vi "GetMicronArgs.vi"(8 "error in (no error)":errorcluster) -> (0 "error out":errorcluster, 3 "Micron Args":T1)   [LabVIEW 2019, in "MicronServer.lvlib" / "ServiceBase.lvclass"]
uses:
  ServiceBase.lvclass
  Typedefs/Micron Args.ctl
  <vilib>/SLL Toolkit/SLL String/_SubVIs/1D String Array to String.vi
  <vilib>/SLL Toolkit/SLL String/SLL String.lvlib
  <vilib>/regexp/Match Regular Expression.xnode
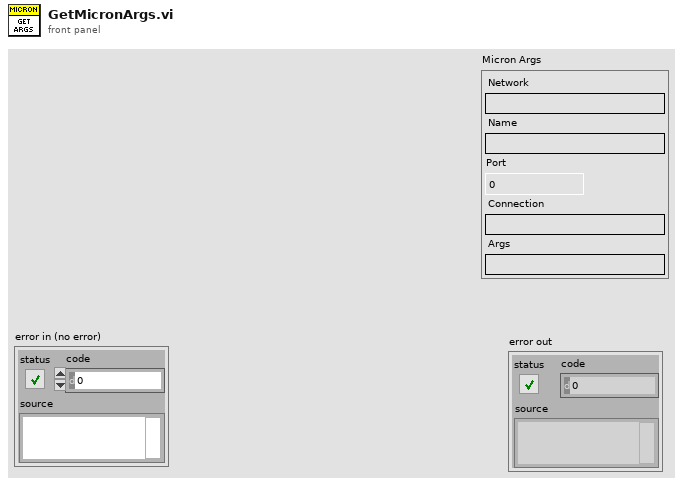
[diagram p1: front panel]
types:
  T1 = typedef "MicronServer.lvlib/ServiceBase.lvclass/Micron Args.ctl" = cluster{"Network":string, "Name":string, "Port":i32, "Connection":string, "Args":string}
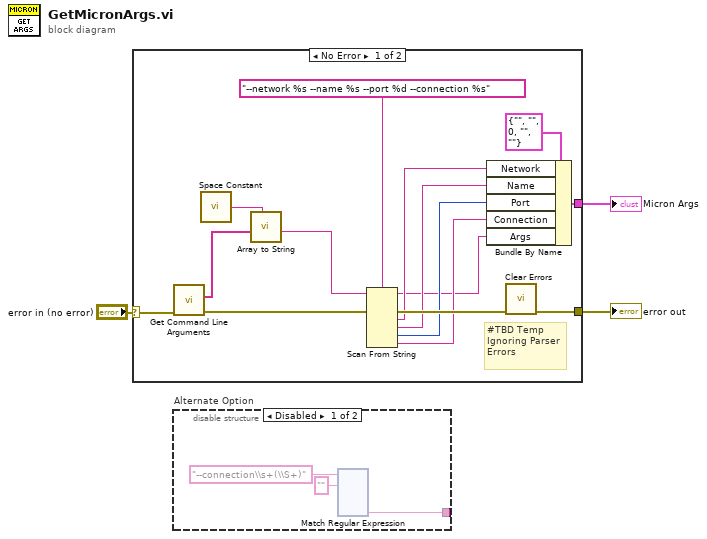
[diagram p0: block diagram]
diagram:
  n1 = case shown="No Error" "error in (no error)" {
    selector: "error in (no error)" -> [w18 w19]
    tunnel: [w4 w19] -> w2
    tunnel: [w5 _] -> w1
    frame No Error {
      # "#TBD Temp \nIgnoring Parser Errors"
      n2 = call <vilib>:"Get Command Line Arguments.vi"("error in (no error)"=w18) -> ("error out"=w15:errorcluster, "arguments"=w17:string[])  [unwired: 8 in, 1 out]
      n3 = call <vilib>:"Space Constant.vi"() -> ("String"=w16:string)
      n4 = call-poly <vilib>:"Array to String.vi"("Delimiter (,)"=w16, "1D Array[]"=w17) -> ("String"=w14:string)  [unwired: 6 in]
      n5 = Scan From String(format string="--network %s --name %s --port %d --connection %s", input string=w14, error in=w15) -> (remaining string=w6:string, error out=w13:errorcluster, output 1=w10:string, output 2=w9:string, output 3=w8:i32, output 4=w7:string)  [unwired: 5 in, 1 out]
      n6 = Bundle By Name(cluster=T1 {"Network"="", "Name"="", "Port"=0, "Connection"="", "Args"=""} ("Micron Args"), "Network"=w10, "Name"=w9, "Port"=w8, "Connection"=w7, "Args"=w6) -> (w5:T1)
      n7 = call <vilib>:"Clear Errors.vi"("error in (no error)"=w13) -> ("error out"=w4:errorcluster)  [unwired: 5 in, 1 out]
    }
    frame Error {
    }
  }
  "error out" <- w2
  "Micron Args" <- w1
  n8 = disable-structure "Alternate Option" shown="Disabled" {
    disable-tunnel: [w21 _] -> _
    frame Disabled {
      n9 = xnode "Match Regular Expression"("input string"="--connection\\s+(\\S+)", "regular expression"="") -> ("submatch 1"=w21:string)  [unwired: 4 in, 5 out]
    }
    frame Enabled {
    }
  }
